vi "Resubmit Folder as different Charge States.vi"() -> ()   [LabVIEW 2010]
uses:
  <vilib>/Utility/file.llb/Write To Spreadsheet File (string).vi
panel:
  in  "CNM Contract Name":string="cnm40004"
  in  "Expected Walltime":dbl=172800.0 format="%<%H:%M:%S>t"
  out "# Electrons":i32
  in  "Desired Net Charge":i32[](array[numeric])=[-2, -1, 1, 2]
  in  "New DIrectory":path=path "D:/Ab-initio/VASP Calcs/2D_Grain Boundaries/Batch38_20130927"
  in  "Original Directory":path=path "D:/Ab-initio/VASP Calcs/2D_Grain Boundaries/Batch37_20130925"
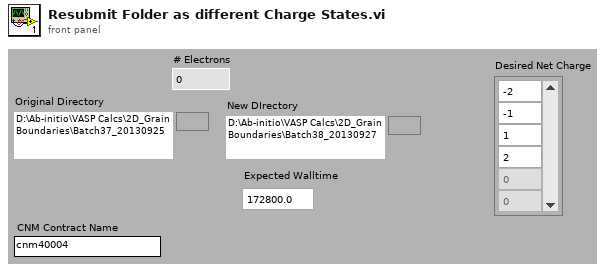
[diagram p1: front panel]
types:
  T1 = cluster{"Email at Beginning?":bool, "Email at End?":bool, "Email when aborted?":bool}
  T2 = cluster{"Number of Nodes":i32, "Processors per node":i32}
  T3 = cluster{"Structure Name":string, "Lattice vector a":dbl[], "Lattice vector b":dbl[], "Lattice vector c":dbl[], "Atoms Array":cluster{"Atom Name":string, "Positions (Direct)":dbl[][], "Positions (Cartesian)":dbl[][]}[], "# of atoms":i32}
  T4 = cluster{"Atom Name":string, "Positions (Direct)":dbl[][], "Positions (Cartesian)":dbl[][]}[]
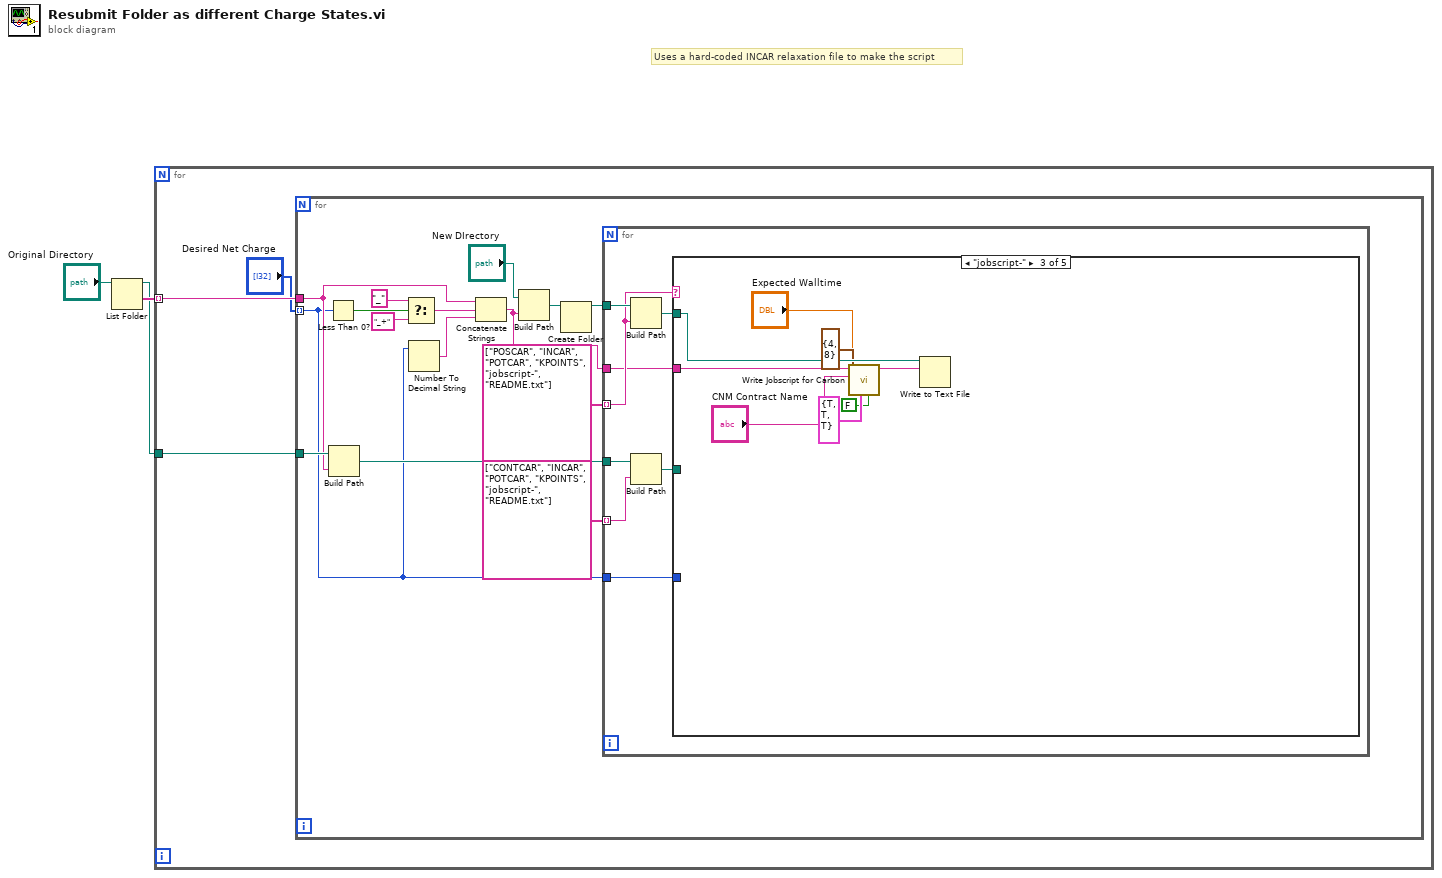
[diagram p0: block diagram]
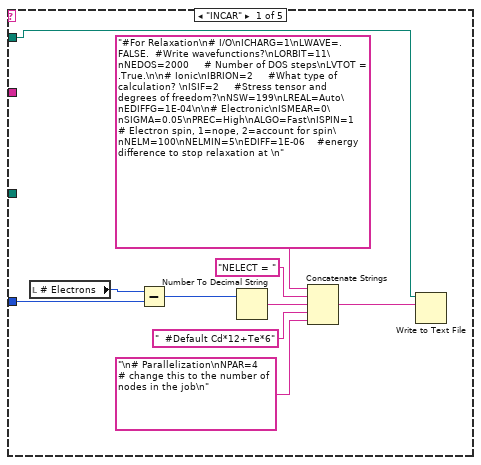
[diagram p2: hidden frame]
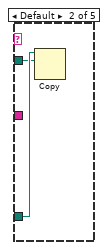
[diagram p3: hidden frame]
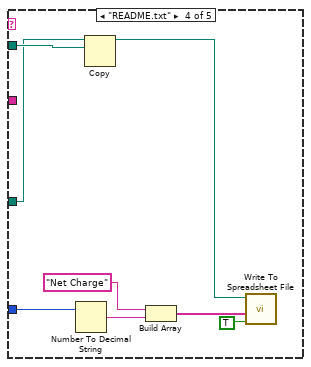
[diagram p4: hidden frame]
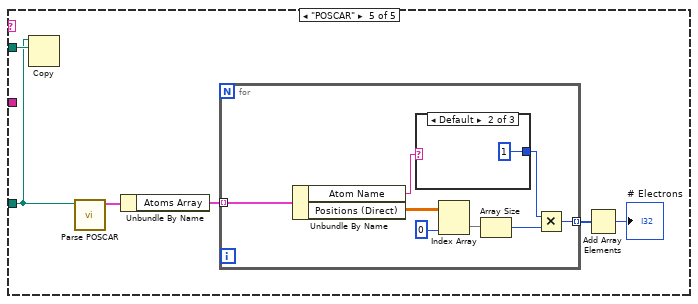
[diagram p5: hidden frame]
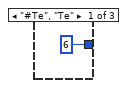
[diagram p6: hidden frame]
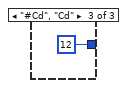
[diagram p7: hidden frame]
diagram:
  # "Uses a hard-coded INCAR relaxation file to make the script"
  n1 = List Folder(path="Original Directory") -> (path out=w1:path, folder names=w2:string[])  [unwired: 3 in, 2 out]
  n2 = for {
    tunnel: w2 -> [w5] mode=indexing
    tunnel: w1 -> [w6]
    n3 = for {
      tunnel: w6 -> [w21]
      tunnel: w5 -> [w14]
      tunnel: "Desired Net Charge" -> [w12] mode=indexing
      n4 = Less Than 0?(x=w12) -> (x < 0?=w11:bool)
      n5 = Build Path(base path=w21, name or relative path=w14) -> (appended path=w18:path)
      n6 = Select(t="_" ("string"), s=w11, f="_+" ("string")) -> (s? t:f=w8:string)
      n7 = Number To Decimal String(number=w12) -> (decimal integer string=w13:string)  [unwired: 1 in]
      n8 = Concatenate Strings(w14, w8, w13) -> (w7:string)
      n9 = Build Path(base path="New DIrectory", name or relative path=w7) -> (appended path=w19:path)
      n10 = Create Folder(path (use dialog)=w19) -> (created path=w17:path)  [unwired: 2 in, 2 out]
      n11 = for {
        tunnel: w18 -> [w29]
        tunnel: w17 -> [w26]
        tunnel: string[] ["CONTCAR", "INCAR", "POTCAR", "KPOINTS", "jobscript-", "README.txt"] -> [w28] mode=indexing
        tunnel: string[] ["POSCAR", "INCAR", "POTCAR", "KPOINTS", "jobscript-", "README.txt"] -> [w24] mode=indexing
        tunnel: w12 -> [w23]
        tunnel: w7 -> [w22]
        n12 = Build Path(base path=w26, name or relative path=w24) -> (appended path=w25:path)
        n13 = Build Path(base path=w29, name or relative path=w28) -> (appended path=w27:path)
        n14 = case shown="\"jobscript-\"" w24 {
          tunnel: w27 -> [_ w41 _ w56 w60]
          tunnel: w25 -> [w39 w40 w48 w57 w63]
          tunnel: w23 -> [w31 _ _ w53 _]
          tunnel: w22 -> [_ _ w47 _ _]
          frame "INCAR" {
            n15 = local read "# Electrons"() -> (w32:i32)
            n16 = Subtract(x=w32, y=w31) -> (x-y=w30:i32)
            n17 = Number To Decimal String(number=w30) -> (decimal integer string=w37:string)  [unwired: 1 in]
            n18 = Concatenate Strings("#For Relaxation\n# I/O\nICHARG=1\nLWAVE=.FALSE.  #Write wavefunctions?\nLORBIT=11\nNEDOS=2000     # Number of DOS steps\nLVTOT = .True.\n\n# Ionic\nIBRION=2     #What type of calculation? \nISIF=2     #Stress tensor and degrees of freedom?\nNSW=199\nLREAL=Auto\nEDIFFG=1E-04\n\n# Electronic\nISMEAR=0\nSIGMA=0.05\nPREC=High\nALGO=Fast\nISPIN=1     # Electron spin, 1=nope, 2=account for spin\nNELM=100\nNELMIN=5\nEDIFF=1E-06    #energy difference to stop relaxation at \n" ("text"), "NELECT = " ("string"), w37, "  #Default Cd*12+Te*6" ("string"), "\n# Parallelization\nNPAR=4     # change this to the number of nodes in the job\n" ("text")) -> (w33:string)
            n19 = Write to Text File(file (use dialog)=w39, text=w33) -> ()  [unwired: 2 in, 3 out]
          }
          frame Default {
            n20 = Copy(10:w40, 11:w41) -> ()  [unwired: 3 in, 3 out]
          }
          frame "jobscript-" {
            n21 = call "Write Jobscript for Carbon.vi"("Load VTST for NEB?"=FALSE, "Email?"=T1 {"Email at Beginning?"=TRUE, "Email at End?"=TRUE, "Email when aborted?"=TRUE}, "Expected Walltime"="Expected Walltime", "Nodes and Processors"=T2 {"Number of Nodes"=4, "Processors per node"=8}, "CNM Contract Name"="CNM Contract Name", "Submitname on Carbon"=w47) -> ("Jobscript"=w49:string)  [unwired: 5 in]
            n22 = Write to Text File(file (use dialog)=w48, text=w49) -> ()  [unwired: 2 in, 3 out]
          }
          frame "README.txt" {
            n23 = Number To Decimal String(number=w53) -> (decimal integer string=w52:string)  [unwired: 1 in]
            n24 = Copy(10:w57, 11:w56) -> (3:w50:path)  [unwired: 3 in, 2 out]
            n25 = Build Array("Net Charge", w52) -> (w51:string[])
            n26 = call-poly <vilib>:"Write To Spreadsheet File.vi"("append to file? (new file:F)"=TRUE, "1D data"=w51, "file path (dialog if empty)"=w50) -> ()  [unwired: 5 in, 1 out]
          }
          frame "POSCAR" {
            n27 = Copy(10:w63, 11:w60) -> ()  [unwired: 3 in, 3 out]
            n28 = call "Parse POSCAR.vi"("POSCAR File"=w60) -> ("Structure"=w59:T3)  [unwired: 7 in, 3 out]
            n29 = Unbundle By Name(w59) -> ("Atoms Array"=w61:T4)
            n30 = for {
              tunnel: w61 -> [w71] mode=indexing
              tunnel: [w66] -> w62 mode=indexing
              n31 = Unbundle By Name(w71) -> ("Atom Name"=w65:string, "Positions (Direct)"=w70:dbl[][])
              n32 = case shown="Default" w65 {
                tunnel: [6 ("x") 1 ("x") 12 ("x")] -> w64
                frame "#Te", "Te" {
                }
                frame Default {
                }
                frame "#Cd", "Cd" {
                }
              }
              n33 = Index Array(array=w70, index (col)=0 ("disabled index (col)")) -> (element=w68:dbl[])  [unwired: 1 in]
              n34 = Array Size(array=w68) -> (size(s)=w67:i32)
              n35 = Multiply(x=w64, y=w67) -> (x*y=w66:i32)
            }
            n36 = Add Array Elements(numeric array=w62) -> (sum=→"# Electrons":i32)
          }
        }
      }
    }
  }
